vi "Configure Event Search (Peak).vi"(5 "Peak Excursion (20)":dbl=20.0, 7 "Peak Threshold (-20)":dbl=-20.0, 8 "error in (no error)":errorcluster, 9 "Maximum Peaks (1)":dbl=1.0, 10 "Source Channel (0: Math 1)":i32(ring) items=["Math 1", "Math 2", "Math 3", "Math 4", "Function 1", "Function 2", "Function 3", "Function 4", "FFT"], 11 "VISA resource name":refnum<visa-resource-name>) -> (0 "error out":errorcluster, 3 "VISA resource name out":refnum<visa-resource-name>)   [LabVIEW 2017, in "Agilent 2000 3000 X-Series.lvlib"]
doc: "Configures the event search of Peak.\n\nNotes:\nThis VI is not supported by EDUX1052A/G, DSOX1202A/G, DSOX1204A/G models.\nThis VI preforms a frequency peak search on the selected FFT math function waveform.\nSo an FFT math function must be configured and enabled before calling this VI.\nIf an enabled FFT math function is not selected as the source a -221, \"Settings conflict\"\nerror will be produced.\nBefore calling this VI:\n1. Call <b>Configure Math Function Characteristics </b>.vi with 5: FFT as the Math Operation\n2. Call <b>Configure Math Function Source </b>.vi with one of 0-3: Channel 1-4 selected for Signal Source 1\n3. Call <b>Configure Math Function (FFT) </b>.vi with the desired parameters\n4. Call <b>Configure Event Search Characteristics </b> with Enable Event Search set to True and Event Search Type set to Peak"
uses:
  Agilent 2000 3000 X-Series.lvlib
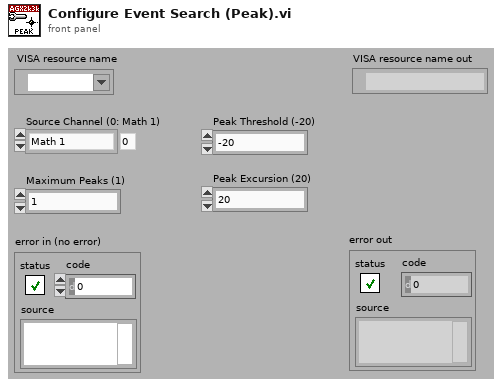
[diagram p1: front panel]
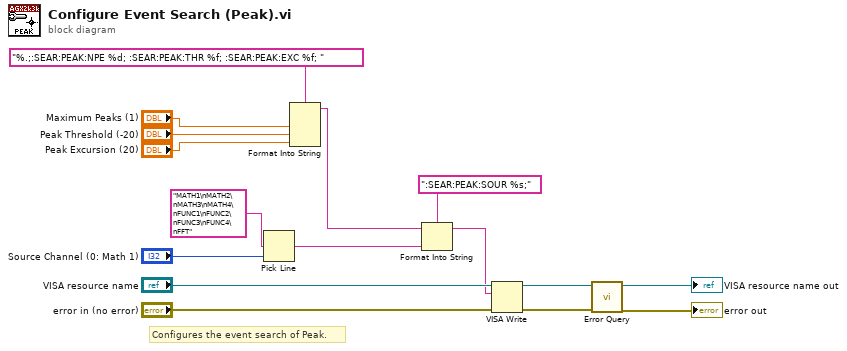
[diagram p0: block diagram]
diagram:
  # "Configures the event search of Peak."
  n1 = Pick Line(multi-line string="MATH1\nMATH2\nMATH3\nMATH4\nFUNC1\nFUNC2\nFUNC3\nFUNC4\nFFT", line index="Source Channel (0: Math 1)") -> (output string=w6:string)  [unwired: 1 out]
  n2 = Format Into String(format string="%.;:SEAR:PEAK:NPE %d; :SEAR:PEAK:THR %f; :SEAR:PEAK:EXC %f; ", "Maximum Peaks (1)", "Peak Threshold (-20)", "Peak Excursion (20)") -> (resulting string=w1:string)  [unwired: 2 in, 1 out]
  n3 = Format Into String(format string=":SEAR:PEAK:SOUR %s;", initial string=w1, w6) -> (resulting string=w10:string)  [unwired: 1 in, 1 out]
  n4 = VISA Write(VISA resource name="VISA resource name", write buffer=w10, error in (no error)="error in (no error)") -> (VISA resource name out=w14:refnum<visa-resource-name>, error out=w13:errorcluster)  [unwired: 1 out]
  n5 = call "Error Query.vi"("error in (no error)"=w13, "VISA resource name"=w14) -> ("error out"=→"error out":errorcluster, "VISA resource name out"=→"VISA resource name out":refnum<visa-resource-name>)  [unwired: 8 out]
